vi "get Session Prefix.vi"(7 "Session - Root":refnum<class "Session - Root.lvclass">) -> (8 "Session Prefix":string)   [LabVIEW 2020, in "Session - Root.lvclass"]
uses:
  <userlib>/_Session Fwk/Session - Root.lvclass
  <userlib>/_Session Fwk/Session - Root.lvclass/Session - Root.ctl
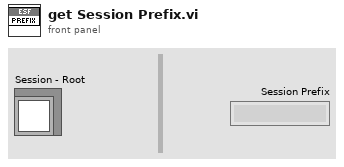
[diagram p1: front panel]
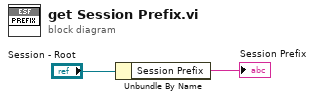
[diagram p0: block diagram]
diagram:
  n1 = Unbundle By Name("Session - Root") -> ("Session Prefix"=→"Session Prefix":string)
